vi "Set 1D Array Double Complex.vi"(5 "use temporary file? (F)":bool, 7 "column vector?":bool, 8 "error in":errorcluster, 9 "value":cdb[](array[numeric]), 10 "variable name":string, 11 "GOLPI ref. in":T1={"pipe handle"={"lv_proc.dll file path"=path "", "process instance handle"=[], "debug mode"=FALSE, "debug data"=[]}, "fast read timeout [ms]"=500, "fast read settle time [ms]"=10, "fast read to multiple [ms]"=1, "max elements per input line"=100, "slow read timeout [ms]"=5000, "stdin double format specifier"="%_16e", "max elements per stdout output column"=100, "console mode bitstream"=FALSE, "bitstream first read timeout [ms]"=1000, "bitstream read timeout [ms]"=50, "struct transfer possible"=FALSE, "matlab mode"=FALSE}) -> (0 "error out":errorcluster, 3 "GOLPI ref. out":T1={"pipe handle"={"lv_proc.dll file path"=path "", "process instance handle"=[], "debug mode"=FALSE, "debug data"=[]}, "fast read timeout [ms]"=500, "fast read settle time [ms]"=10, "fast read to multiple [ms]"=1, "max elements per input line"=100, "slow read timeout [ms]"=5000, "stdin double format specifier"="%_16e", "max elements per stdout output column"=100, "console mode bitstream"=FALSE, "bitstream first read timeout [ms]"=1000, "bitstream read timeout [ms]"=50, "struct transfer possible"=FALSE, "matlab mode"=FALSE})   [LabVIEW 2020, in "GOLPI library.lvlib"]
doc: "Part of polymorph Set Variable.vi"
uses:
  GOLPI library.lvlib
  GOLPI reference Type Def.ctl
  Pipe Handle.ctl
  LV Process library.lvlib
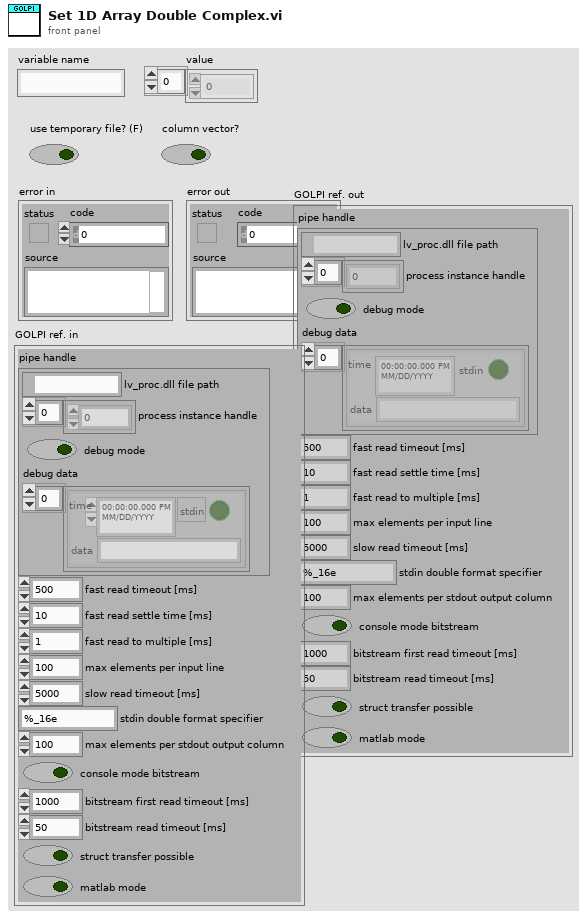
[diagram p1: front panel]
types:
  T1 = typedef "GOLPI library.lvlib/GOLPI reference Type Def.ctl" = cluster{"pipe handle":T2, "fast read timeout [ms]":u32, "fast read settle time [ms]":u32, "fast read to multiple [ms]":u32, "max elements per input line":u32, "slow read timeout [ms]":u32, "stdin double format specifier":string, "max elements per stdout output column":u32, "console mode bitstream":bool, "bitstream first read timeout [ms]":u32, "bitstream read timeout [ms]":u32, "struct transfer possible":bool, "matlab mode":bool}
  T2 = typedef "LV Process library.lvlib/Pipe Handle.ctl" = cluster{"lv_proc.dll file path":path, "process instance handle":u32[], "debug mode":bool, "debug data":cluster{"time":timestamp, "stdin":bool, "data":string}[]}
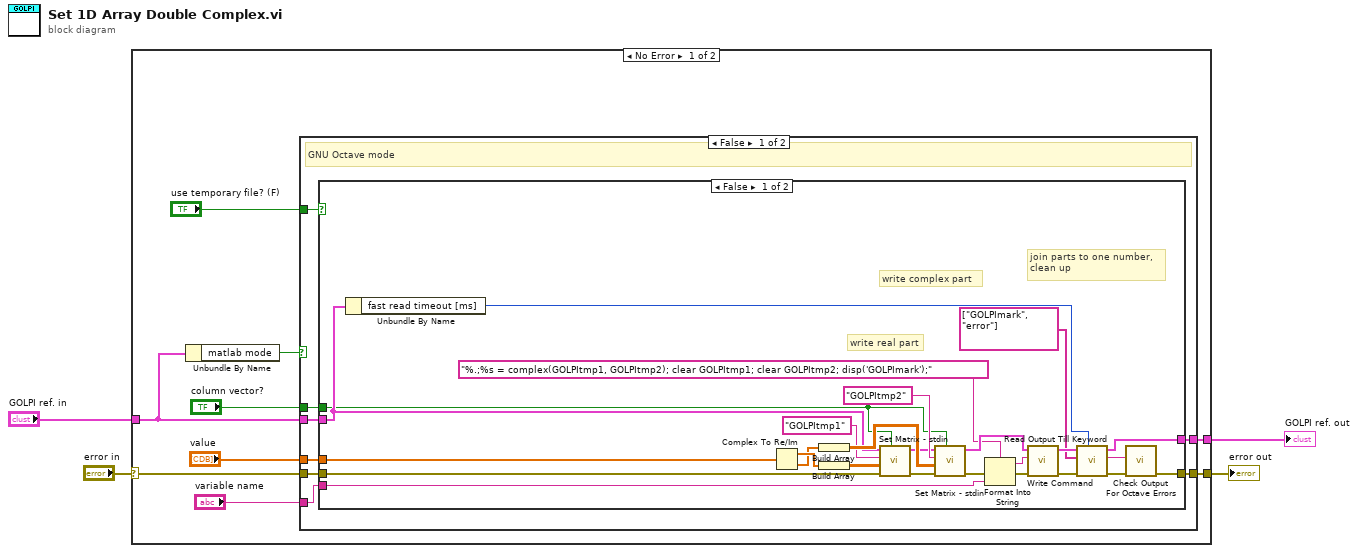
[diagram p0: block diagram]
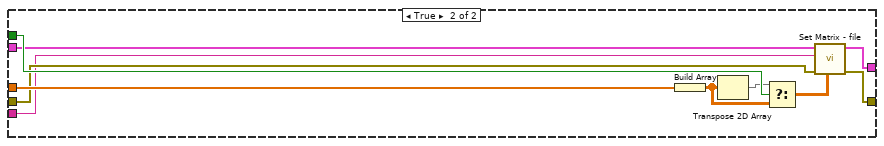
[diagram p2: hidden frame]
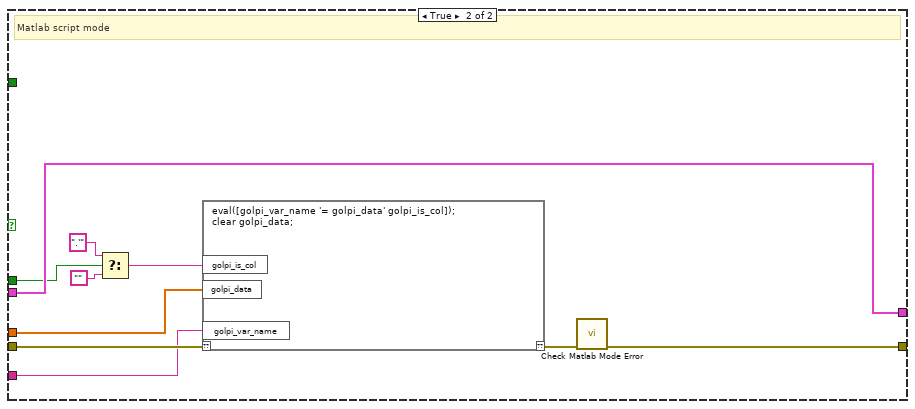
[diagram p3: hidden frame]
diagram:
  n1 = case shown="No Error" "error in" {
    selector: "error in" -> [w13 w69]
    tunnel: [w10 w69] -> w4
    tunnel: "GOLPI ref. in" -> [w6 w68]
    tunnel: [w11 w68] -> w1
    frame No Error {
      n2 = Unbundle By Name(w6) -> ("matlab mode"=w5:bool)
      n3 = case shown="False" w5 {
        tunnel: w13 -> [w21 w67]
        tunnel: "variable name" -> [w20 w66]
        tunnel: [w19 w64] -> w11
        tunnel: [w18 w58] -> w10
        tunnel: w6 -> [w17 w64]
        tunnel: "use temporary file? (F)" -> [w16 _]
        tunnel: "column vector?" -> [w15 w61]
        tunnel: "value" -> [w14 w65]
        frame False {
          # "GNU Octave mode"
          n4 = case shown="False" w16 {
            tunnel: w21 -> [w47 w54]
            tunnel: w20 -> [w34 w51]
            tunnel: [w30 w52] -> w19
            tunnel: [w28 w53] -> w18
            tunnel: w17 -> [w26 w55]
            tunnel: w15 -> [w23 w56]
            tunnel: w14 -> [w22 w57]
            frame False {
              # "join parts to one number,\nclean up"
              # "write complex part"
              # "write real part"
              n5 = Unbundle By Name(w26) -> ("fast read timeout [ms]"=w25:u32)
              n6 = Complex To Re/Im(x + iy=w22) -> (x=w45:dbl[], y=w42:dbl[])
              n7 = Build Array(w42) -> (w43:dbl[][])
              n8 = Build Array(w45) -> (w46:dbl[][])
              n9 = call "Set Matrix - stdin.vi"("swap dimensions? (F)"=w23, "error in"=w47, "value"=w46, "variable name"="GOLPItmp1", "GOLPI ref. in"=w26) -> ("error out"=w41:errorcluster, "GOLPI ref. out"=w40:T1)  [unwired: 5 in]
              n10 = call "Set Matrix - stdin.vi"("swap dimensions? (F)"=w23, "error in"=w41, "value"=w43, "variable name"="GOLPItmp2", "GOLPI ref. in"=w40) -> ("error out"=w39:errorcluster, "GOLPI ref. out"=w38:T1)  [unwired: 5 in]
              n11 = Format Into String(format string="%.;%s = complex(GOLPItmp1, GOLPItmp2); clear GOLPItmp1; clear GOLPItmp2; disp('GOLPImark');" ("command"), error in=w39, w34) -> (resulting string=w36:string, error out=w37:errorcluster)  [unwired: 1 in]
              n12 = call "Write Command.vi"("error in"=w37, "command"=w36, "GOLPI ref. in"=w38) -> ("error out"=w33:errorcluster, "GOLPI ref. out"=w32:T1)  [unwired: 7 in]
              n13 = call "Read Output Till Keyword.vi"("timeout [ms]"=w25, "error in"=w33, "keywords"=string[] ["GOLPImark", "error"], "GOLPI ref. in"=w32) -> ("error out"=w29:errorcluster, "read buffer"=w27:string, "GOLPI ref. out"=w30:T1)  [unwired: 4 in, 1 out]
              n14 = call "Check Output For Octave Errors.vi"("error in"=w29, "read buffer"=w27) -> ("error out"=w28:errorcluster)  [unwired: 9 in]
            }
            frame True {
              n15 = Build Array(w57) -> (w49:cdb[][])
              n16 = Transpose 2D Array(2D array=w49) -> (transposed array=w48:cdb[][])
              n17 = Select(t=w48, s=w56, f=w49) -> (s? t:f=w50:cdb[][])
              n18 = call "Set Matrix - file.vi"("cmplx double array"=w50, "error in (no error)"=w54, "variable name"=w51, "GOLPI ref. in"=w55) -> ("error out"=w53:errorcluster, "GOLPI ref. out"=w52:T1)  [unwired: 6 in]
            }
          }
        }
        frame True {
          # "Matlab script mode"
          n19 = Select(t=".'", s=w61, f="") -> (s? t:f=w60:string)
          n20 = script code="eval([golpi_var_name '= golpi_data' golpi_is_col]);\nclear golpi_data;"("??"=w67, "golpi_var_name"=w66, "golpi_data"=w65, "golpi_is_col"=w60) -> ("??"=w59:errorcluster)
          n21 = call "Check Matlab Mode Error.vi"("error in"=w59) -> ("error out"=w58:errorcluster)  [unwired: 10 in]
        }
      }
    }
    frame Error {
    }
  }
  "error out" <- w4
  "GOLPI ref. out" <- w1
